vi "Teleop.vi"(10 "Match Info":T1={"Autonomous Elapsed Seconds"=0.0, "TeleOp Elapsed Seconds"=0.0, "Disabled Elapsed Seconds"=0.0, "Visited Autonomous"=FALSE, "Visited TeleOp"=FALSE, "Visited Disabled"=FALSE, "Autonomous Settings"={"Autonomous Style"=enum."Independent", "VI Refnum"=refnum}}, 11 "Call Context":T2) -> ()   [LabVIEW 2017]
doc: "This VI is called for each TeleOp packet received from the DS where the robot is not disabled. It is often used to read from the joysticks and update I/O or to update setpoints for timed control loops. It should complete and return within 20 milliseconds or it may miss DS packets."
uses:
  <vilib>/Rock Robotics/WPI/DriverStation/WPI_DriverStationDerivedRobotMode.ctl
  <vilib>/Rock Robotics/WPI/DriverStation/WPI_DriverStationMatch Info.ctl
  <vilib>/Rock Robotics/WPI/Utilities/WPI_GetSetVariantRefNum.vi
  <vilib>/Rock Robotics/Network Tables/NT Write Boolean Array.vi
  <vilib>/Rock Robotics/Network Tables/NT Write Numeric Array.vi
  <vilib>/Rock Robotics/Network Tables/NT Read Boolean.vi
  <vilib>/Rock Robotics/Network Tables/NT Read Number.vi
  Robot Global Data.vi
  <vilib>/Rock Robotics/Network Tables/NT Write Number.vi
panel:
  out "Sample Slider 0":dbl(slide) scale=0.0..5.0
  out "Sample Boolean 1":bool
  out "Sample Boolean 0":bool
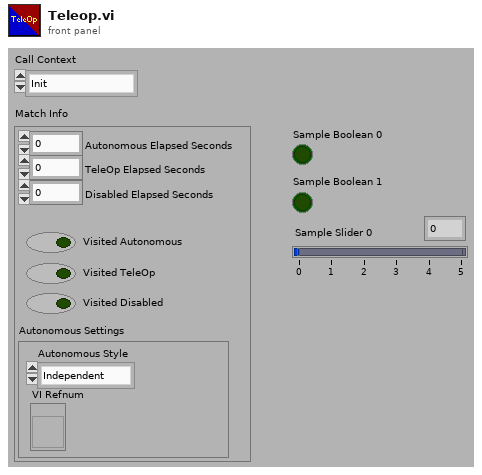
[diagram p1: front panel]
types:
  T1 = typedef "WPI_DriverStationMatch Info.ctl" = cluster{"Autonomous Elapsed Seconds":dbl, "TeleOp Elapsed Seconds":dbl, "Disabled Elapsed Seconds":dbl, "Visited Autonomous":bool, "Visited TeleOp":bool, "Visited Disabled":bool, "Autonomous Settings":cluster{"Autonomous Style":enum16{"Iterative", "Independent"}, "VI Refnum":refnum<vi>}}
  T2 = typedef "WPI_DriverStationDerivedRobotMode.ctl" = enum16{"Init", "Execute", "Stop"}
  T3 = typedef "WPI_RobotDriveDevRef.ctl" = cluster{"DevStatus":errorcluster, "Motors[]":T4[], "Square Inputs":bool, "Max Output":dbl}
  T4 = typedef "WPI_MotorControlDeviceRef.ctl" = cluster{"DeviceStatus":errorcluster, "Type":T5, "PWM":cluster{"PWM Channel":T6, "DeadBand":T7}, "CAN":cluster{"Device Number":u8, "SetOutput VI Ref":variant, "GetOutput VI Ref":variant, "Enable VI Ref":variant, "Disable VI Ref":variant, "Data":variant}, "Invert":bool, "DIO PWM":cluster{"PWM \"Enable\" Channel":T6, "DIOChannel":T8, "PWM Rate":dbl}}
  T5 = typedef "WPI_MotorControlType.ctl" = enum16{"PWM", "CAN", "DIO PWM"}
  T6 = typedef "FPGA_DIOPWMChannel.ctl" = enum8{"PWM 0", "PWM 1", "PWM 2", "PWM 3", "PWM 4", "PWM 5", "PWM 6", "PWM 7", "PWM 8", "PWM 9", "PWM MXP 0", "PWM MXP 1", "PWM MXP 2", "PWM MXP 3", "PWM MXP 4", "PWM MXP 5", "PWM MXP 6", "PWM MXP 7", "PWM MXP 8", "PWM MXP 9", "Invalid"}
  T7 = typedef "WPI_PWMDeadband.ctl" = cluster{"Name":string, "maxPositivePwm":i32, "minPositivePwm":i32, "centerPwm":i32, "maxNegativePwm":i32, "minNegativePwm":i32, "angularRange":u16}
  T8 = typedef "FPGA_DIOChannel.ctl" = enum8{"DIO 0", "DIO 1", "DIO 2", "DIO 3", "DIO 4", "DIO 5", "DIO 6", "DIO 7", "DIO 8", "DIO 9", "DIO MXP 0", "DIO MXP 1", "DIO MXP 2", "DIO MXP 3", "DIO MXP 4", "DIO MXP 5", "DIO MXP 6", "DIO MXP 7", "DIO MXP 8", "DIO MXP 9", "DIO MXP 10", "DIO MXP 11", "DIO MXP 12", "DIO MXP 13", "DIO MXP 14", "DIO MXP 15", "SPI Port CS1", "SPI Port CS2", "SPI Port CS3", "SPI Port MISO", "SPI Port MOSI", "Invalid"}
  T9 = typedef "WPI_JoystickDevRef.ctl" = cluster{"Device":T10}
  T10 = typedef "WPI_JoystickDeviceEnum.ctl" = enum16{"USB 0", "USB 1", "USB 2", "USB 3", "USB 4", "USB 5"}
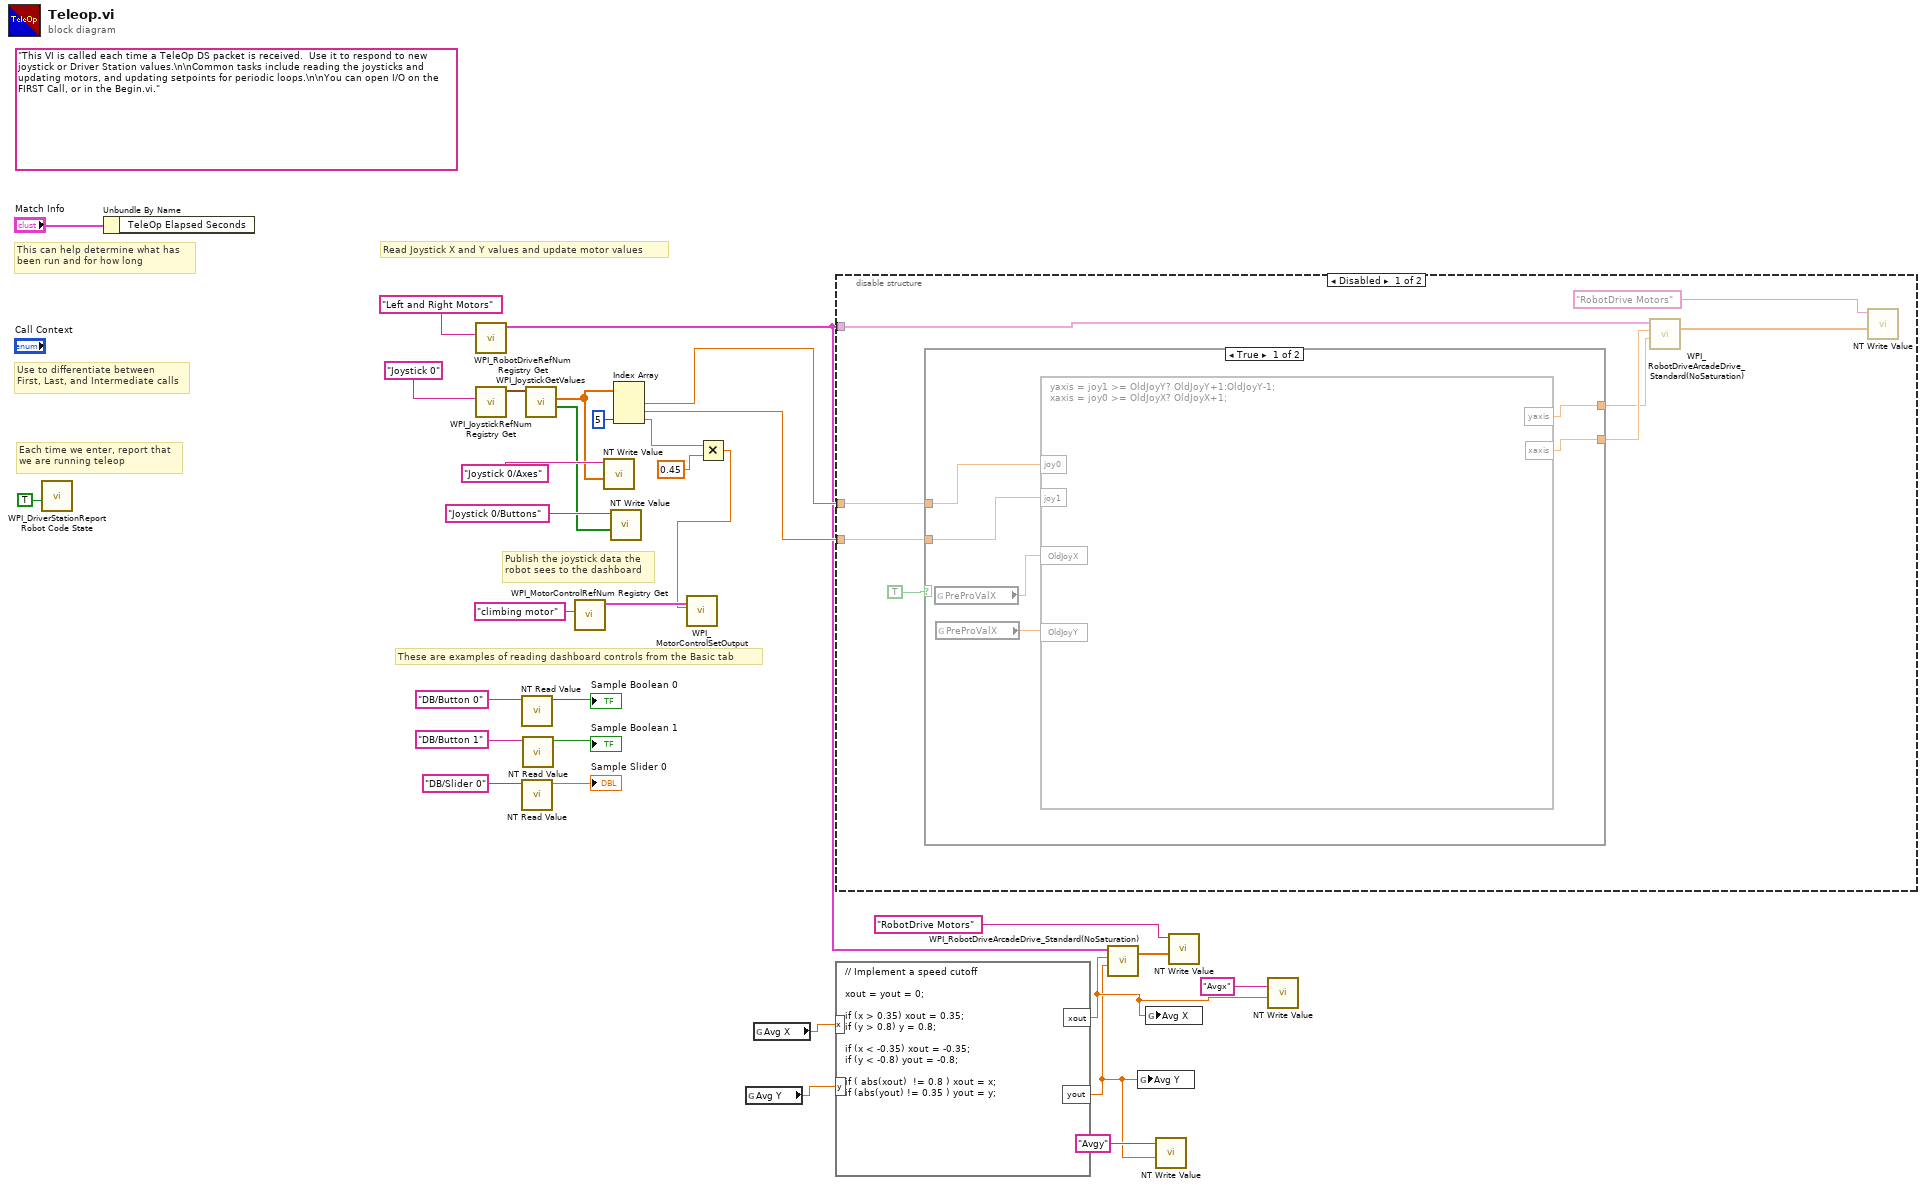
[diagram p0: block diagram]
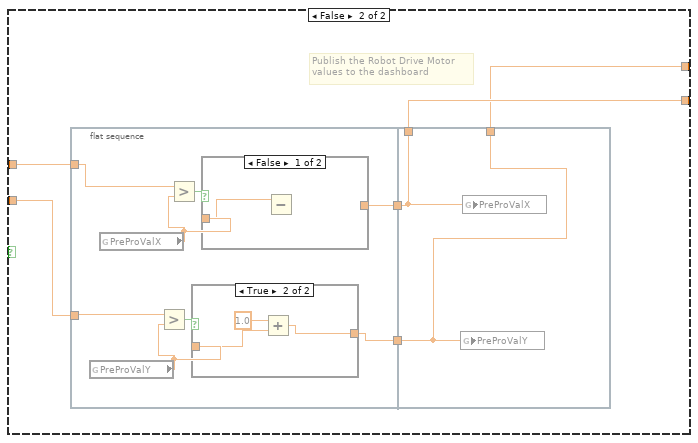
[diagram p2: hidden frame]
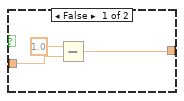
[diagram p3: hidden frame]
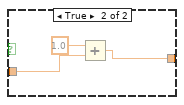
[diagram p4: hidden frame]
diagram:
  (unwired) "This VI is called each time a TeleOp DS packet is received.  Use it to respond to new joystick or Driver Station values.\n\nCommon tasks include reading the joysticks and updating motors, and updating setpoints for periodic loops.\n\nYou can open I/O on the FIRST Call, or in the Begin.vi."
  # "These are examples of reading dashboard controls from the Basic tab"
  # "Publish the joystick data the\nrobot sees to the dashboard"
  # "Each time we enter, report that\nwe are running teleop"
  # "Use to differentiate between\nFirst, Last, and Intermediate calls"
  # "This can help determine what has\nbeen run and for how long"
  # "Read Joystick X and Y values and update motor values"
  n1 = call <vilib>:"WPI_DriverStationReport Robot Code State.vi"("TeleOp"=TRUE ("Autonomous")) -> ()  [unwired: 10 in, 1 out]
  n2 = Unbundle By Name("Match Info") -> ()  [unwired: 1 out]
  n3 = call <vilib>:"WPI_RobotDriveRefNum Registry Get.vi"("refnum name"="Left and Right Motors") -> ("RobotDriveDevRef"=w13:T3)  [unwired: 1 in, 9 out]
  n4 = call <vilib>:"WPI_JoystickRefNum Registry Get.vi"("refnum name"="Joystick 0") -> ("JoystickDevRef"=w29:T9)  [unwired: 1 in, 9 out]
  n5 = call-poly <vilib>:"NT Read Value.vi"("Name"="DB/Button 0" ("refnum name")) -> ("Boolean"=→"Sample Boolean 0":bool)  [unwired: 9 in, 1 out]
  n6 = call-poly <vilib>:"NT Read Value.vi"("Name"="DB/Slider 0" ("refnum name")) -> ("Numeric"=→"Sample Slider 0":dbl)  [unwired: 9 in, 1 out]
  n7 = call-poly <vilib>:"NT Read Value.vi"("Name"="DB/Button 1" ("refnum name")) -> ("Boolean"=→"Sample Boolean 1":bool)  [unwired: 9 in, 1 out]
  n8 = call <vilib>:"WPI_JoystickGetValues.vi"("JoystickDevRef"=w29) -> ("Buttons"=w24:bool[], "Axes"=w25:dbl[])  [unwired: 6 in, 3 out]
  n9 = call <vilib>:"WPI_MotorControlRefNum Registry Get.vi"("refnum name"="climbing motor") -> ("MotorControlDevRef"=w2:T4)  [unwired: 9 in, 1 out]
  n10 = call-poly <vilib>:"NT Write Value.vi"("Numeric Array"=w25, "Name"="Joystick 0/Axes") -> ()  [unwired: 9 in, 1 out]
  n11 = call-poly <vilib>:"NT Write Value.vi"("Boolean Array"=w24, "Name"="Joystick 0/Buttons") -> ()  [unwired: 9 in, 1 out]
  n12 = Index Array(array=w25, index #3=5 ("index")) -> (element #1=w17:dbl, element #2=w16:dbl, element #3=w5:dbl)  [unwired: 2 in]
  n13 = Multiply(x=w5, y=0.45) -> (x*y=w1:dbl)
  n14 = call <vilib>:"WPI_MotorControlSetOutput.vi"("Output"=w1, "MotorControlDevRef"=w2) -> ()  [unwired: 7 in, 3 out]
  n15 = global read "Robot Global Data.vi" "Avg Y"() -> (w11:dbl)
  n16 = global read "Robot Global Data.vi" "Avg X"() -> (w12:dbl)
  n17 = formula code="// Implement a speed cutoff\n\nxout = yout = 0;\n\nif (x > 0.35) xout = 0.35; \nif (y > 0.8) y = 0.8;\n\nif (x < -0.35) xout = -0.35;\nif (y < -0.8) yout = -0.8;\n\nif ( abs(xout)  != 0.8 ) xout = x;\nif (abs(yout) != 0.35 ) yout = y;"("x"=w12, "y"=w11) -> ("xout"=w9:dbl, "yout"=w7:dbl)
  n18 = disable-structure shown="Disabled" {
    disable-tunnel: w13 -> [w40 _]
    disable-tunnel: w17 -> [w36 _]
    disable-tunnel: w16 -> [w35 _]
    frame Disabled {
      n19 = case shown="True" TRUE ("Boolean") {
        tunnel: [w45 w50] -> w37
        tunnel: w36 -> [w44 w49]
        tunnel: w35 -> [w43 w48]
        tunnel: [w46 w47] -> w34
        frame True {
          n20 = global read "Robot Global Data.vi" "PreProValX"() -> (w42:dbl)
          n21 = global read "Robot Global Data.vi" "PreProValX"() -> (w41:dbl)
          n22 = formula code="yaxis = joy1 >= OldJoyY? OldJoyY+1:OldJoyY-1;\nxaxis = joy0 >= OldJoyX? OldJoyX+1;"("joy1"=w43, "joy0"=w44, "OldJoyX"=w42, "OldJoyY"=w41) -> ("yaxis"=w46:dbl, "xaxis"=w45:dbl)
        }
        frame False {
          # "Publish the Robot Drive Motor\nvalues to the dashboard"
          n23 = flat-sequence {
            tunnel: w49 -> [w60]
            tunnel: [w57] -> w52
            tunnel: w48 -> [w54]
            tunnel: [w53] -> w51
            tunnel: w52 -> [w72]
            tunnel: [w72] -> w50
            tunnel: w51 -> [w71]
            tunnel: [w71] -> w47
            frame #0 {
              n24 = global read "Robot Global Data.vi" "PreProValY"() -> (w56:dbl)
              n25 = global read "Robot Global Data.vi" "PreProValX"() -> (w58:dbl)
              n26 = Greater?(x=w54, y=w56) -> (0:w55:bool)
              n27 = Greater?(x=w60, y=w58) -> (0:w59:bool)
              n28 = case shown="True" w55 {
                tunnel: w56 -> [w63 w66]
                tunnel: [w61 w64] -> w53
                frame False {
                  n29 = Subtract(x=1.0, y=w63) -> (x-y=w61:dbl)
                }
                frame True {
                  n30 = Add(x=1.0, y=w66) -> (x+y=w64:dbl)
                }
              }
              n31 = case shown="False" w59 {
                tunnel: w58 -> [w67 w70]
                tunnel: [_ w68] -> w57
                frame False {
                  n32 = Subtract(x=w67) -> ()  [unwired: 1 in, 1 out]
                }
                frame True {
                  n33 = Add(x=1.0, y=w70) -> (x+y=w68:dbl)
                }
              }
            }
            frame #1 {
              n34 = global write "Robot Global Data.vi" "PreProValY"(w71) -> ()
              n35 = global write "Robot Global Data.vi" "PreProValX"(w72) -> ()
            }
          }
        }
      }
      n36 = call <vilib>:"WPI_RobotDriveArcadeDrive_Standard(NoSaturation).vi"("Y axis value"=w34, "X axis value"=w37, "RobotDriveDevRef"=w40) -> ("Motor Values"=w39:dbl[])  [unwired: 1 in, 7 out]
      n37 = call-poly <vilib>:"NT Write Value.vi"("Numeric Array"=w39, "Name"="RobotDrive Motors") -> ()  [unwired: 9 in, 1 out]
    }
    frame Enabled {
    }
  }
  n38 = call <vilib>:"WPI_RobotDriveArcadeDrive_Standard(NoSaturation).vi"("Y axis value"=w7, "X axis value"=w9, "RobotDriveDevRef"=w13) -> ("Motor Values"=w14:dbl[])  [unwired: 1 in, 7 out]
  n39 = global write "Robot Global Data.vi" "Avg Y"(w7) -> ()
  n40 = global write "Robot Global Data.vi" "Avg X"(w9) -> ()
  n41 = call-poly <vilib>:"NT Write Value.vi"("Numeric"=w7, "Name"="Avgy") -> ()  [unwired: 9 in, 1 out]
  n42 = call-poly <vilib>:"NT Write Value.vi"("Numeric Array"=w14, "Name"="RobotDrive Motors") -> ()  [unwired: 9 in, 1 out]
  n43 = call-poly <vilib>:"NT Write Value.vi"("Numeric"=w9, "Name"="Avgx") -> ()  [unwired: 9 in, 1 out]
